vi "LIA Filter and Decimate.vi"(0 "I":fxp<+/-,36,2> format="%.35g", 1 "filter in":T1 {"mSRate_QSettings"."source" items=["Coef a/k"=0, "Coef b/v"=7, "Input"=1, "Output"=2, "Multiplicand"=3, "Product"=4, "Sum"=5, "Delay"=6, "Gain"=8]}, 5 "Q":fxp<+/-,36,2> format="%.35g", 11 "input valid":bool, 12 "Decimation":i32) -> (4 "I Decimated":dbl, 6 "Q Decimated":dbl, 15 "output valid":bool)   [LabVIEW 2017]
uses:
  <vilib>/addons/Digital Filter Design/_Objects.llb/DFD Filter Obj.ctl
  <vilib>/addons/Digital Filter Design/_Objects.llb/DFD Filter Coef.ctl
  <vilib>/addons/Digital Filter Design/_Objects.llb/DFD Filter Structure Type Selector.ctl
  <vilib>/addons/Digital Filter Design/_Objects.llb/dfd_Internal Quantization Settings.ctl
  <vilib>/addons/Digital Filter Design/_Objects.llb/dfd_Internal Quantization Srcs.ctl
  <vilib>/addons/Digital Filter Design/_Objects.llb/DFD Coef Norm Type.ctl
  <vilib>/addons/Digital Filter Design/Process.llb/DFD Filtering (PtByPt).vi
  <vilib>/addons/Digital Filter Design/NI_DigFilterLicensed.lvlib
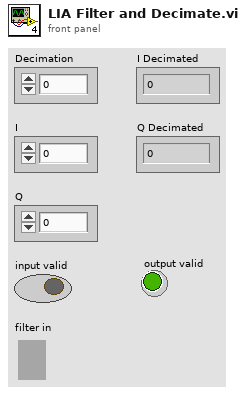
[diagram p1: front panel]
types:
  T1 = typedef "NI_DigFilterLicensed.lvlib/DFD Filter Obj.ctl" = cluster{"mSRate_Fs":dbl, "mSRate_Version":string, "mSRate_Comments":string, "mSRate_OrgCoef":T2, "mSRate_CurCoef":T2, "mSRate_Quantized?":bool, "mSRate_QCoef":T2, "mSRate_QSettings":T4[], "mSRate_Order":i32, "mSRate_Scaling":cluster{"mSRate_ScaleByPowerOf2?":bool, "mSRate_ScaleType":T6}}
  T2 = typedef "NI_DigFilterLicensed.lvlib/DFD Filter Coef.ctl" = cluster{"type":T3, "gain":dbl, "coef a (k)":dbl[], "coef b (v)":dbl[]}
  T3 = typedef "NI_DigFilterLicensed.lvlib/DFD Filter Structure Type Selector.ctl" = enum16{"Undefined", "FIR Direct Form", "FIR Direct Form Transposed", "FIR Symmetric", "FIR Antisymmetric", "IIR Direct Form I", "IIR Direct Form I Transposed", "IIR Direct Form II", "IIR Direct Form II Transposed", "IIR Cascaded Second Order Sections Form I", "IIR Cascaded Second Order Sections Form I Transposed", "IIR Cascaded Second Order Sections Form II", "IIR Cascaded Second Order Sections Form II Transposed", "Lattice Allpass (basic sections)", "Lattice Allpass (one multiplier sections)", "Lattice Allpass (normalized sections)", "Lattice AR (basic sections)", "Lattice AR (one multiplier sections)", "Lattice AR (normalized sections)", "Lattice MA (minimum phase)", "Lattice MA (maximum phase)", "Lattice ARMA (basic sections)", "Lattice ARMA (one multiplier sections)", "Lattice ARMA (normalized sections)"}
  T4 = typedef "NI_DigFilterLicensed.lvlib/dfd_Internal Quantization Settings.ctl" = cluster{"source":T5, "wl":i16, "iwl":i16, "overflow mode":enum16{"Saturation", "Wrap"}, "rounding mode":enum16{"Nearest", "Truncation"}, "signed?":bool}
  T5 = typedef "NI_DigFilterLicensed.lvlib/dfd_Internal Quantization Srcs.ctl" = u16
  T6 = typedef "NI_DigFilterLicensed.lvlib/DFD Coef Norm Type.ctl" = enum16{"No Norm", "Time Domain 1-Norm", "Time Domain 2-Norm", "Time Domain Inf-Norm"}
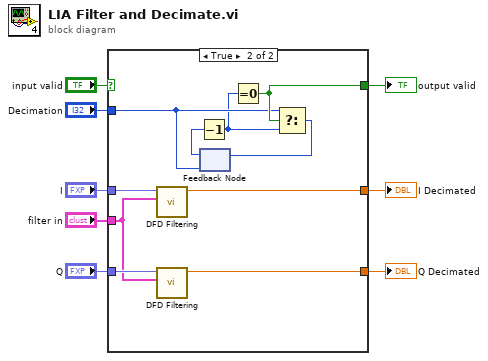
[diagram p0: block diagram]
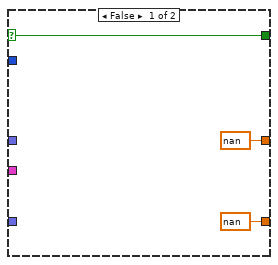
[diagram p2: hidden frame]
diagram:
  n1 = case shown="True" "input valid" {
    selector: "input valid" -> [w9 _]
    tunnel: "I" -> [_ w21]
    tunnel: "Q" -> [_ w20]
    tunnel: "filter in" -> [_ w17]
    tunnel: [nan ("signal out") w19] -> w5
    tunnel: [nan ("signal out") w18] -> w6
    tunnel: [w9 w15] -> w4
    tunnel: "Decimation" -> [_ w13]
    frame False {
    }
    frame True {
      n2 = call-poly <vilib>:"DFD Filtering.vi"("filter"=w17, "signal in"=w21) -> ("signal out"=w19:dbl)  [unwired: 8 in, 1 out]
      n3 = call-poly <vilib>:"DFD Filtering.vi"("filter"=w17, "signal in"=w20) -> ("signal out"=w18:dbl)  [unwired: 8 in, 1 out]
      n4 = feedback #1(w13) -> (w14:i32)
      n5 = Decrement(x=w14) -> (x-1=w12:i32)
      n6 = Equal To 0?(x=w12) -> (x = 0?=w15:bool)
      n7 = Select(t=w13, s=w15, f=w12) -> (s? t:f=w16:i32)
      n8 = feedback-in #1(w16) -> ()
    }
  }
  "Q Decimated" <- w6
  "I Decimated" <- w5
  "output valid" <- w4
